vi "TSCAN_SetChannelCount.vi"(8 "错误输入（无错误）":errorcluster, 10 "Aount":i32, 11 "路径输入":path) -> (0 "错误输出":errorcluster, 3 "路径输出":path, 4 "Set_CAN_Count_Successfully":bool)   [LabVIEW 2019]
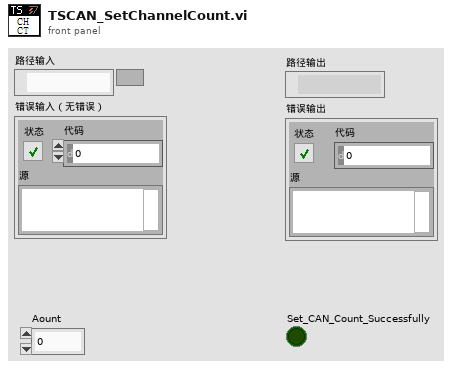
[diagram p1: front panel]
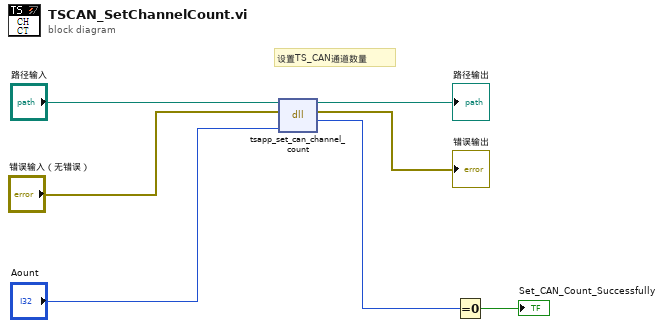
[diagram p0: block diagram]
diagram:
  # "设置TS_CAN通道数量"
  n1 = dll-call lib="PTH2Habs CUsers\nAdministratorDesktopTS_Can通讯PathTSMaster.dll" fn="tsapp_set_can_channel_count"(path in="路径输入", error in="错误输入（无错误）", "Aount"="Aount") -> (path out=→"路径输出":path, error out=→"错误输出":errorcluster, "tsapp_set_can_channel_count"=w4:i32)  [unwired: 2 in]
  n2 = Equal To 0?(x=w4) -> (x = 0?=→"Set_CAN_Count_Successfully":bool)
